vi "Configure Voltage Range.vi"(8 "error in (no error)":errorcluster, 10 "Output Mode (0: Low)":i32(ring) items=["Low", "High"], 11 "VISA resource name":refnum<visa-resource-name>) -> (0 "error out":errorcluster, 3 "VISA resource name out":refnum<visa-resource-name>)   [LabVIEW 2018, in "BK Precision 983X Series.lvlib"]
doc: "Selects between the low or high range of the instrument.\n\nNote: When in high range, maximum output current and current limit will be limited to half."
uses:
  <instrlib>/BK Precision 983X Series/BK Precision 983X Series.lvlib
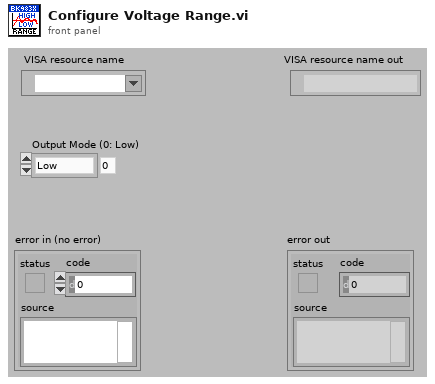
[diagram p1: front panel]
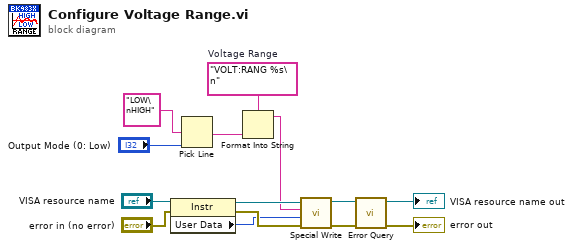
[diagram p0: block diagram]
diagram:
  w2 = "VOLT:RANG %s\n"  # Voltage Range
  n1 = property class="Instr"(reference="VISA resource name", error in="error in (no error)") -> (reference out=w6:refnum<visa-resource-name>, error out=w8:errorcluster, "User Data"=w7:u32)
  n2 = Pick Line(multi-line string="LOW\nHIGH", line index="Output Mode (0: Low)") -> (output string=w3:string)  [unwired: 1 in]
  n3 = Format Into String(format string=w2, w3) -> (resulting string=w1:string)  [unwired: 2 in, 1 out]
  n4 = call <instrlib>:"Special Write.vi"("error in (no error)"=w8, "Delay (0 ms)"=w7, "Input String"=w1, "VISA resource name"=w6) -> ("error out"=w11:errorcluster, "VISA resource name out"=w12:refnum<visa-resource-name>)  [unwired: 6 in]
  n5 = call <instrlib>:"Error Query.vi"("error in (no error)"=w11, "VISA resource name"=w12) -> ("error out"=→"error out":errorcluster, "VISA resource name out"=→"VISA resource name out":refnum<visa-resource-name>)  [unwired: 6 in, 2 out]
